vi "Parallel Executing Test Code.vi"(9 "Test Complete Event":refnum<user-event>, 10 "Positions":u32[](array[numeric]), 11 "MTS Temp Sensor Test in":refnum<class "MTS Memory Test.lvclass">) -> ()   [LabVIEW 2015, in "MTS Memory Test.lvclass"]
uses:
  MTS Memory Test.lvclass
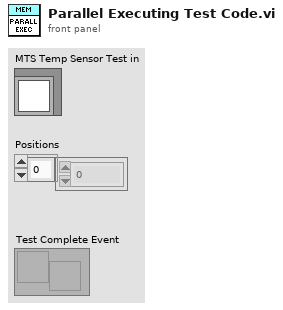
[diagram p1: front panel]
types:
  T1 = cluster{"status":bool, "code":i32, "source":string, "Position":u32}
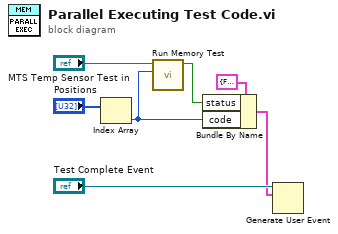
[diagram p0: block diagram]
diagram:
  n1 = Index Array(array="Positions") -> (element=w1:u32)  [unwired: 1 in]
  n2 = call "Run Memory Test.vi"("Position"=w1, "MTS Memory Test in"="MTS Temp Sensor Test in") -> ("Test Passed"=w2:bool)  [unwired: 8 in, 1 out]
  n3 = Bundle By Name(cluster=T1 {"status"=FALSE, "code"=0, "source"="", "Position"=0} ("event data"), "status"=w2, "code"=w1) -> (w3:T1)
  n4 = Generate User Event(user event="Test Complete Event", event data cluster=w3) -> ()  [unwired: 2 in, 2 out]
